vi "Stage Motion Sub VI.vi"() -> ()   [LabVIEW 2009]
uses:
  <vilib>/Instr/_visa.llb/VISA Configure Serial Port (Instr).vi
  <vilib>/Platform/TimedLoop/XDataNode/XDataNode.xnode
  <vilib>/Platform/TimedLoop/XDataNode/loadlvalarms.vi
  <vilib>/Platform/TimedLoop/XDataNode/timing_clust.ctl
  <vilib>/Platform/TimedLoop/XDataNode/nitl_modes.ctl
  <vilib>/Platform/TimedLoop/XDataNode/wakeup.ctl
  <vilib>/Platform/TimedLoop/XDataNode/XDNodeRunTimeDep.lvlib
panel:
  in  "Move to Position 1":bool
  in  "Move to Position 2":bool
  in  "Move to Position 3":bool
  in  "Move to Position 4":bool
  in  "Move to Position 5":bool
  in  "Lower Ch. Cap.":bool
  in  "Dump Beads":bool
  in  "+z":bool
  in  "-z":bool
  in  "z nudge increment (um)":dbl=0.5
  in  "Lower Cap.":bool
  in  "Upper Cap.":bool
  in  "Move to Position":bool
  in  "Set Position":bool
  in  "Position":dbl=1.0 min=1.0 max=10.0 step=1.0
  in  "Saved Stage Positions":dbl[][](array[numeric])=[[1.0, 0.0, 0.0, 0.0], [2.0, 0.0, 0.0, 0.0], [3.0, 0.0, 0.0, 0.0], [4.0, 0.0, 0.0, 0.0], [5.0, 0.0, 0.0, 0.0], [6.0, 0.0, 0.0, 0.0], [7.0, 0.0, 0.0, 0.0], [8.0, 0.0, 0.0, 0.0], [9.0, 0.0, 0.0, 0.0], [10.0, 0.0, 0.0, 0.0]]
  in  "Set Position 1":bool
  in  "Set Position 2":bool
  in  "Set Position 3":bool
  in  "Set Position 4":bool
  in  "Set Position 5":bool
  in  "Position Label 5":string="Lower Channel Cap" caption="5"
  out "Stage Moving":bool
  out "Stage Control Serial Error":errorcluster
  in  "Sample Chamber Stage Serial Port":refnum<visa-resource-name>="ChamberStageCOM4"
  in  "Position 4 Label":string="Dump beads" caption="4"
  in  "Position 3 Label":string="Measurement spot" caption="3"
  in  "Position 2 Label":string="Lower capillary" caption="2"
  in  "Position 1 Label":string="Upper capillary" caption="1"
  in  "Stop All":bool
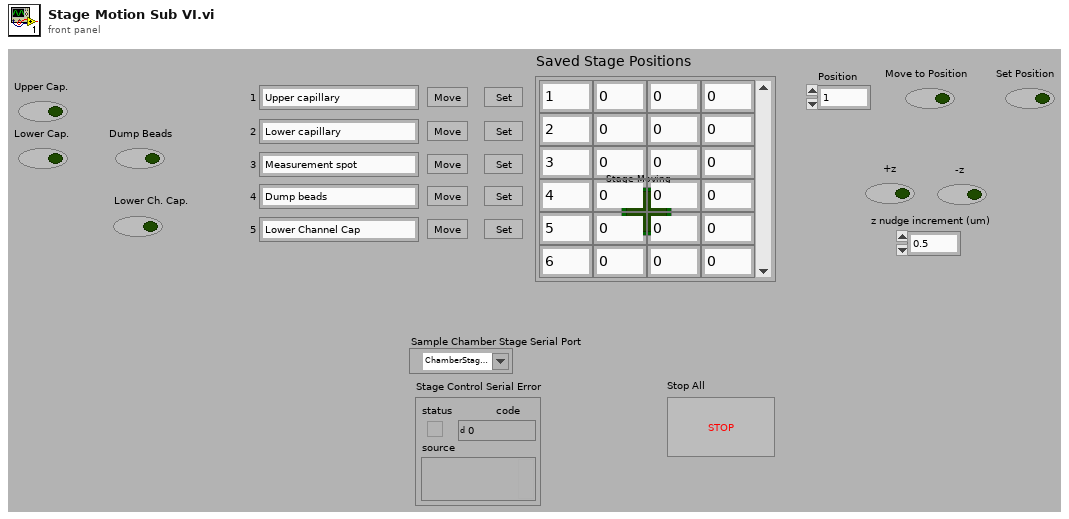
[diagram p1: front panel]
types:
  T1 = typedef "XDNodeRunTimeDep.lvlib/timing_clust.ctl" = cluster{"Expected End [f-1]":u64, "Actual End [f-1]":u64, "Finished Late? [f-1]":bool, "Expected End [i-1]":u64, "Actual End [i-1]":u64, "Finished Late? [i-1]":bool, "Expected Start [i]":u64, "Actual Start [i]":u64, "Expected Start [f]":u64, "Actual Start [f]":u64, "Source Name":string, "Structure Name":string, "Period":i64, "Deadline":i64, "Offset":i64, "Start":i64, "Priority":i32, "Timeout":i32, "Mode":T2, "Wakeup Reason":T3, "Error":errorcluster, "Source Type":string, "Secondary Source Type":string, "Global End Time":u64, "Global Start Time":u64, "Frame Duration":u64, "Iteration Duration":u64, "Assigned CPU":i32, "I/O Scan Engine Mode":u32}
  T2 = typedef "XDNodeRunTimeDep.lvlib/nitl_modes.ctl" = enum32{"No Change", "Process missed periods, maintain original phase", "Discard missed periods, maintain original phase", "Process missed periods, ignore original phase", "Discard missed periods, ignore original phase"}
  T3 = typedef "XDNodeRunTimeDep.lvlib/wakeup.ctl" = enum32{"Normal", "Aborted", "Asynchronous wakeup", "Timing source error", "Timed loop error", "Timeout"}
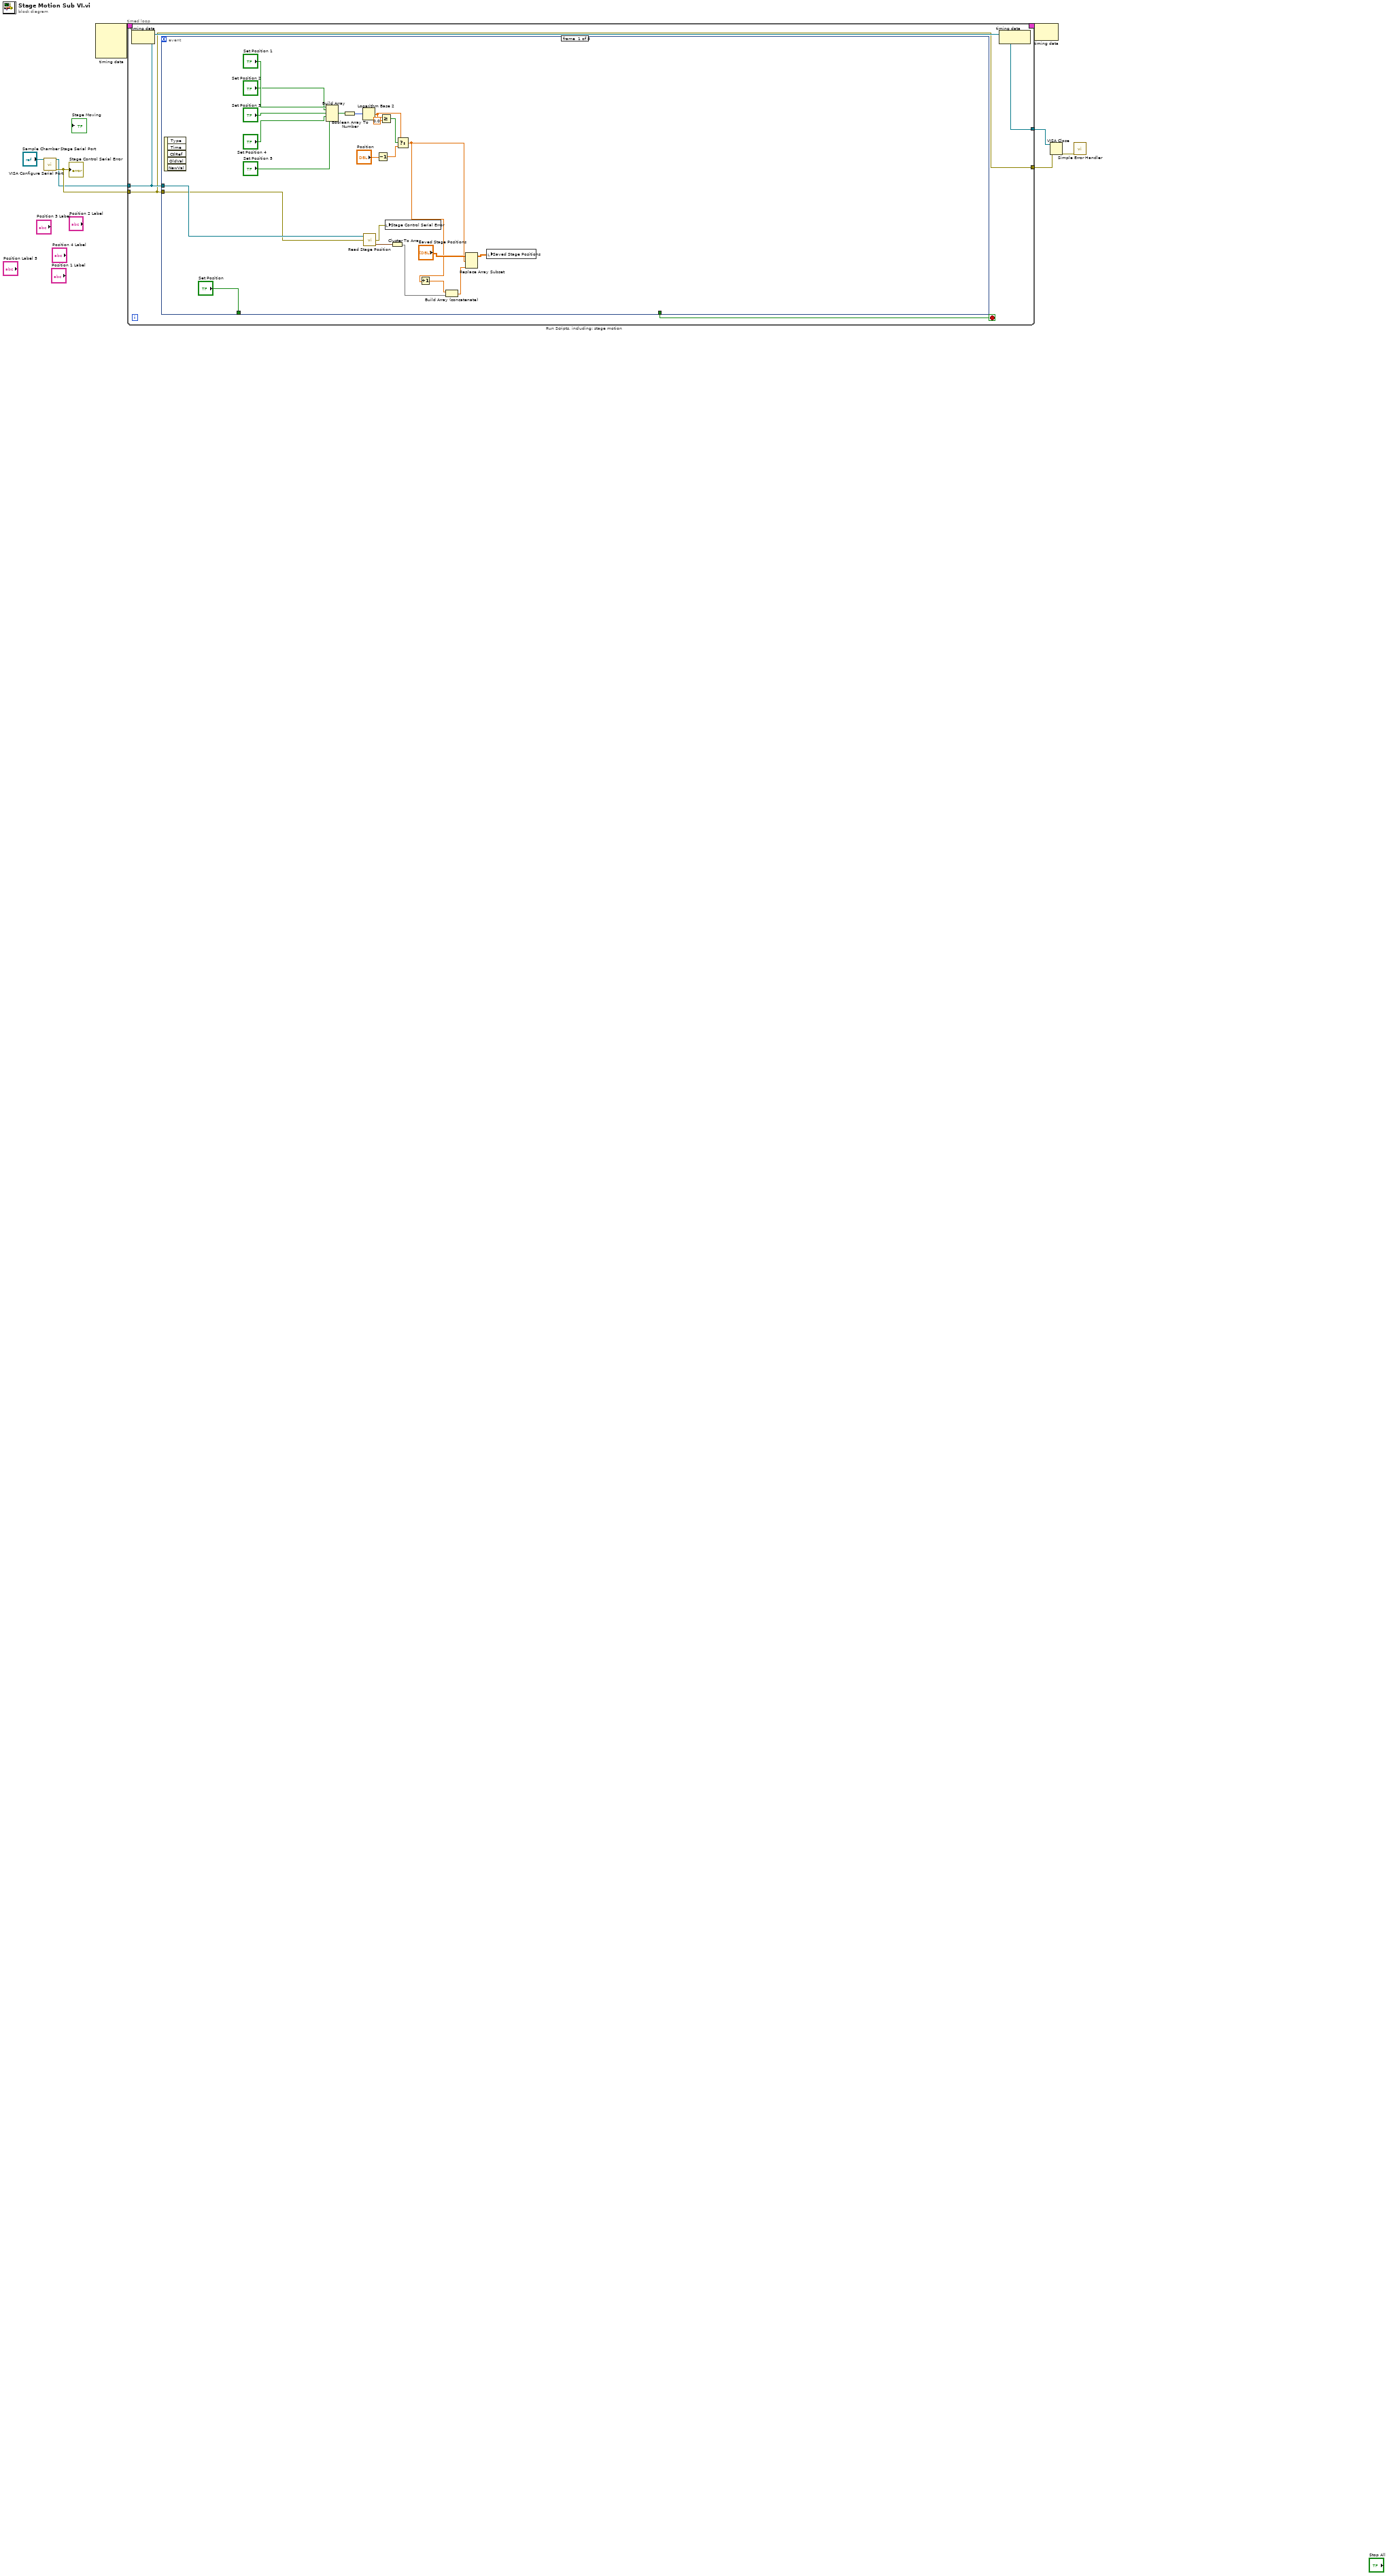
[diagram p0: block diagram]
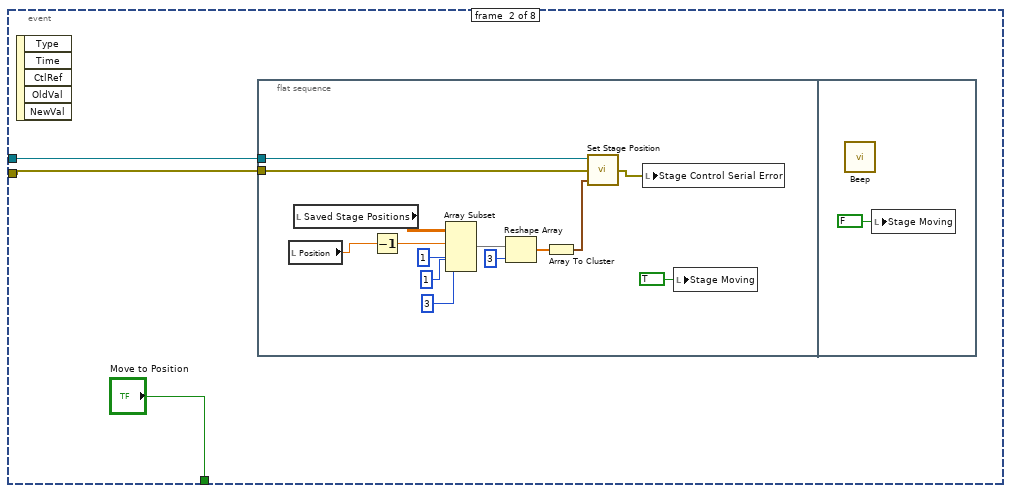
[diagram p2: hidden frame]
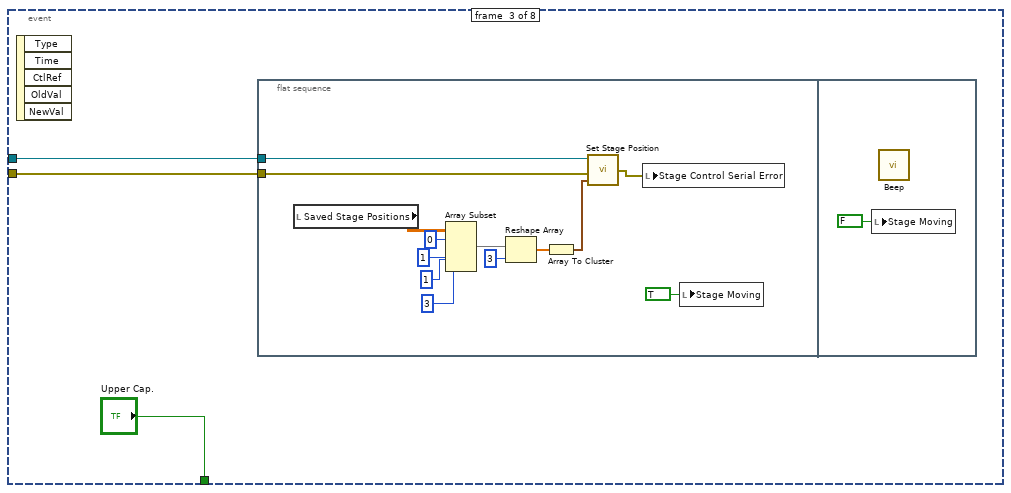
[diagram p3: hidden frame]
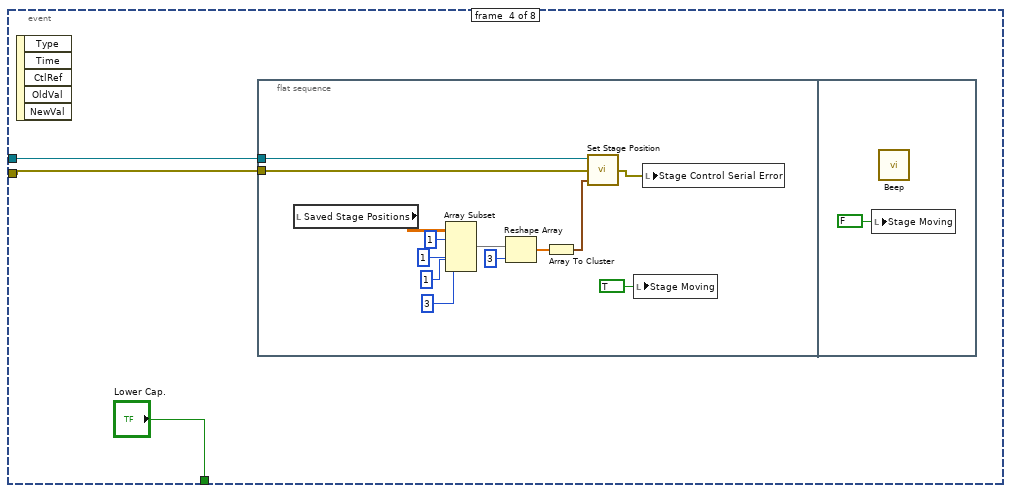
[diagram p4: hidden frame]
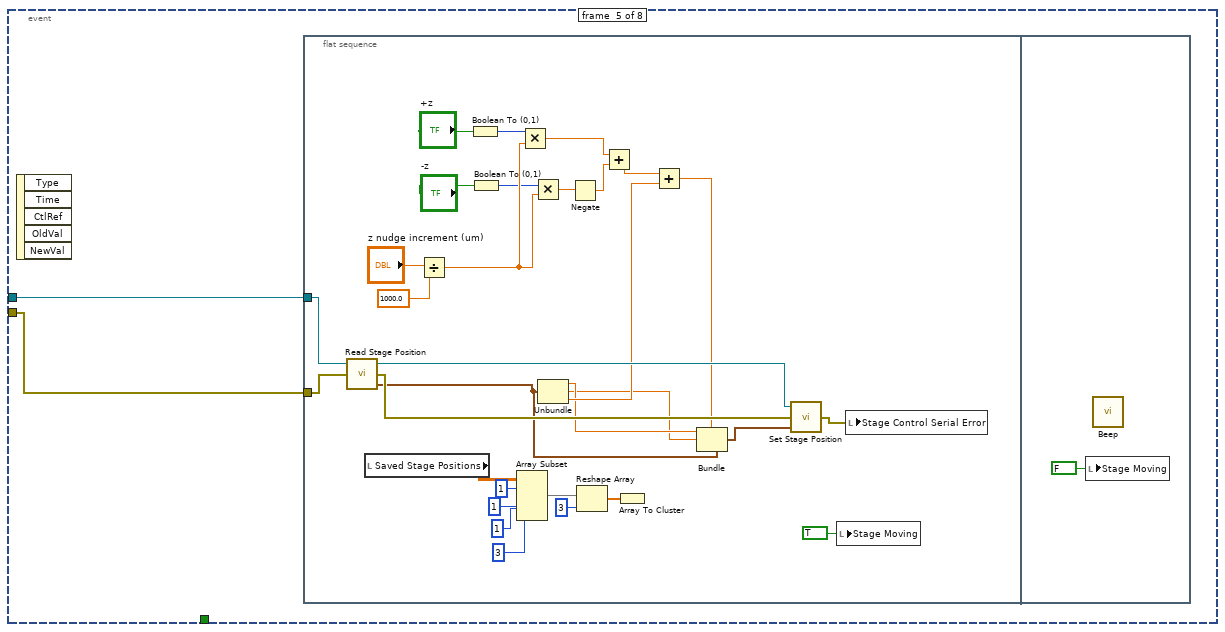
[diagram p5: hidden frame]
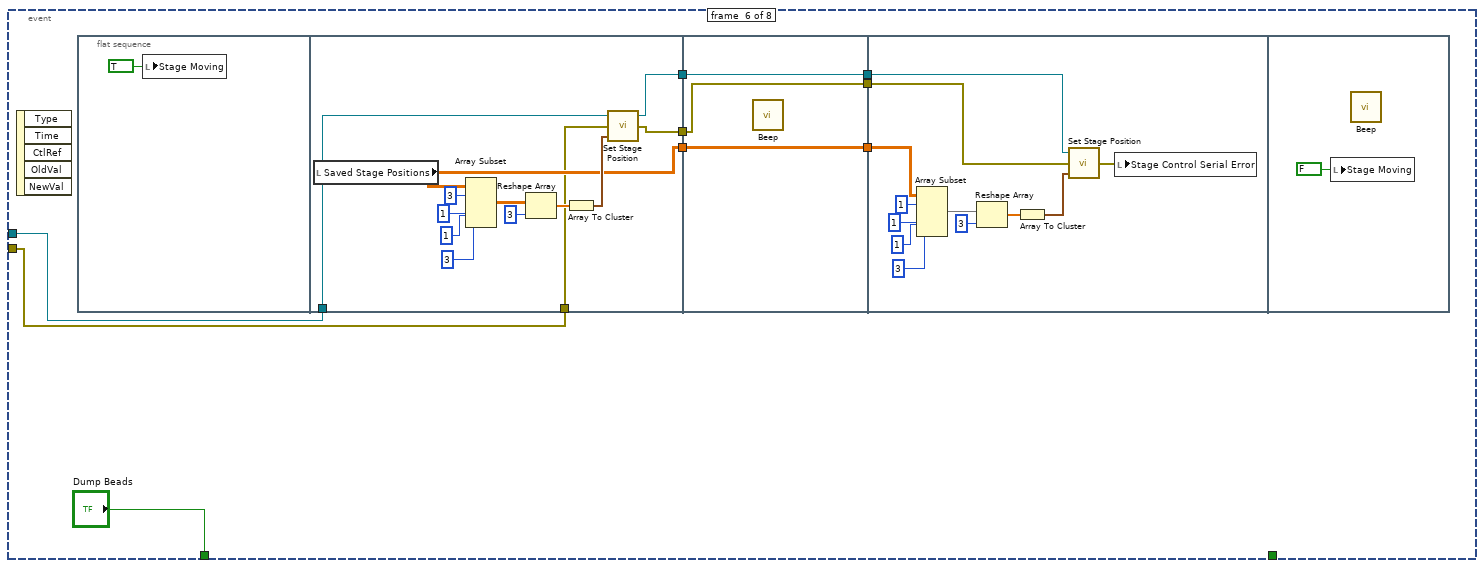
[diagram p6: hidden frame]
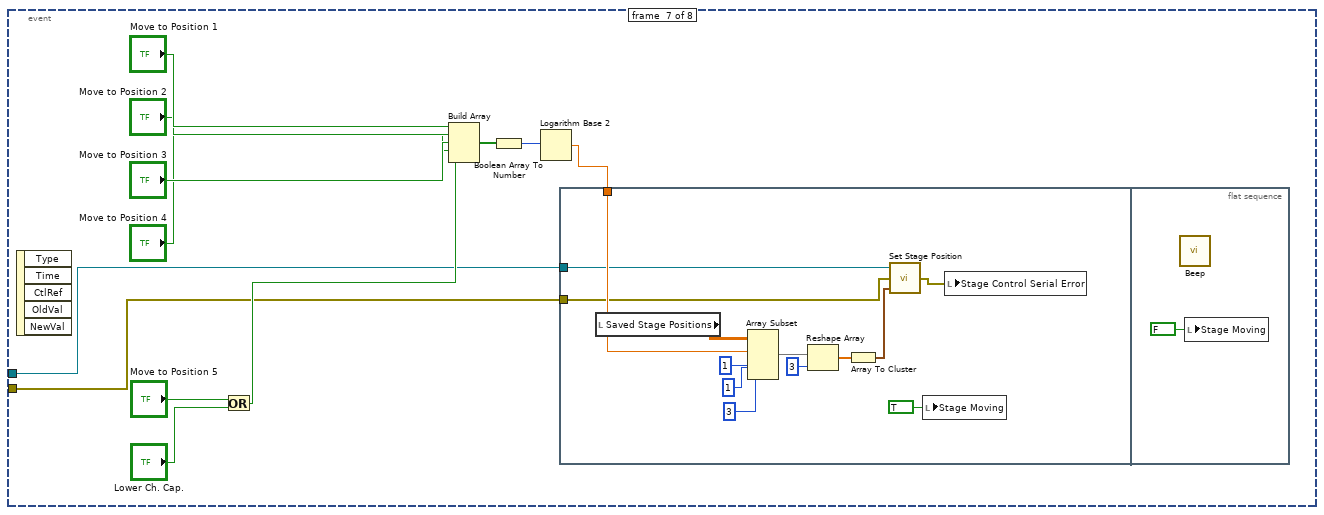
[diagram p7: hidden frame]
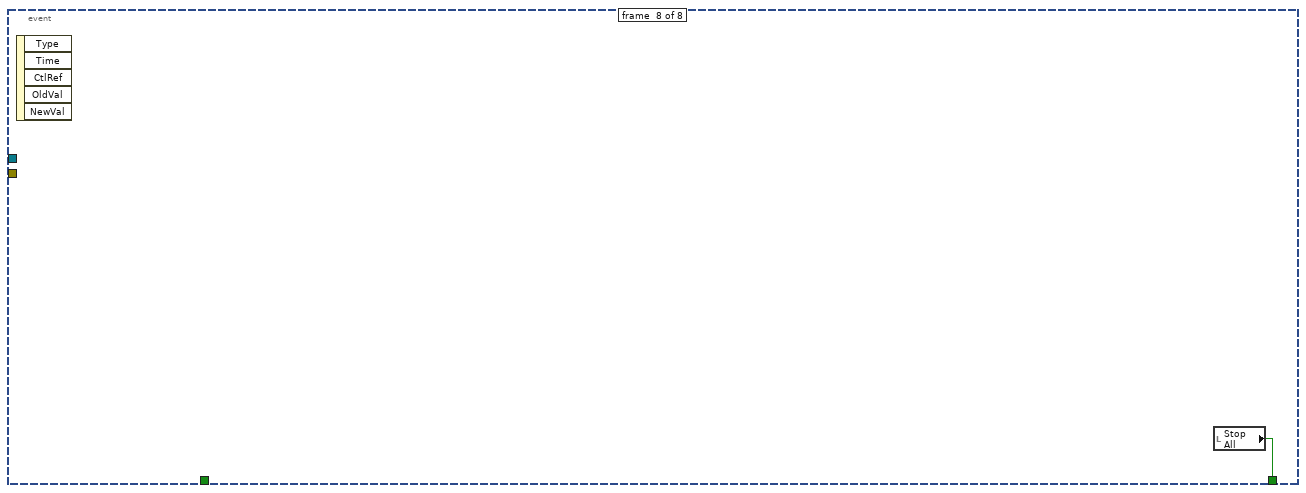
[diagram p8: hidden frame]
diagram:
  n1 = call-poly "VISA Configure Serial Port"("VISA resource name"="Sample Chamber Stage Serial Port") -> ("VISA resource name out"=w3:refnum<visa-resource-name>, "error out"=w4:errorcluster)  [unwired: 5 in, 8 out]
  "Stage Control Serial Error" <- w4
  n2 = node-c288() -> (w8:T1)  [unwired: 4 in]
  n3 = timed-loop "Run Scripts, including: stage motion" {
    tunnel: w4 -> [w9]
    tunnel: w3 -> [w10]
    tunnel: [w10] -> w2
    tunnel: [w9] -> w1
    timing: w8 -> [_]
    timing-out: [_] -> w7
    stop <- w11 stop-if-true
    n4 = node-c288() -> ()  [unwired: 1 in, 1 out]
    n5 = event shown="[7] \"Stop All\": Value Change" {
      selector: _ -> [_ _ _ _ _ _ _ _]
      dyn-events: _ -> [_ _ _ _ _ _ _ _]
      timeout: _ -> [_ _ _ _ _ _ _ _]
      tunnel: ["Set Position" "Move to Position" "Upper Cap." "Lower Cap." _ "Dump Beads" _ _] -> _
      tunnel: [_ _ _ _ _ _ _ w188] -> w11
      tunnel: w9 -> [w29 w37 w55 w72 w89 w123 w162 _]
      tunnel: w10 -> [w30 w38 w56 w73 w90 w124 w163 _]
      event #0 {
        n6 = event-data() -> ()  [unwired: 1 in, 5 out]
        n7 = Build Array("Set Position 1", "Set Position 2", "Set Position 3", "Set Position 4", "Set Position 5") -> (w28:bool[])
        n8 = Boolean Array To Number(Boolean array=w28) -> (number=w27:u32)
        n9 = Logarithm Base 2(1:w27) -> (0:w19:dbl)
        n10 = call "Read Stage Position.vi"("error in"=w29, "VISA resource name in"=w30) -> ("Current Position"=w34:cluster{dbl, dbl, dbl}, "error out"=w33:errorcluster)  [unwired: 2 out]
        n11 = Decrement(x="Position") -> (x-1=w17:dbl)
        n12 = Greater Or Equal?(x=w19, y=0.0) -> (x >= y?=w20:bool)
        n13 = local write "Stage Control Serial Error"(w33) -> ()
        n14 = Cluster To Array(cluster=w34) -> (array=w31:dbl[])
        n15 = Select(t=w19, s=w20, f=w17) -> (s? t:f=w16:dbl)
        n16 = Increment(x=w16) -> (x+1=w15:dbl)
        n17 = Build Array (concatenate)(w15, w31) -> (w14:dbl[])
        n18 = Replace Array Subset(array="Saved Stage Positions", new element=w14, index (row)=w16) -> (w32:dbl[][])  [unwired: 1 in]
        n19 = local write "Saved Stage Positions"(w32) -> ()
      }
      event #1 {
        n20 = event-data() -> ()  [unwired: 1 in, 5 out]
        n21 = flat-sequence {
          tunnel: w38 -> [w41]
          tunnel: w37 -> [w40]
          frame #0 {
            n22 = local read "Position"() -> (w53:dbl)
            n23 = local read "Saved Stage Positions"() -> (w51:dbl[][])
            n24 = Decrement(x=w53) -> (x-1=w50:dbl)
            n25 = Array Subset(array=w51, index (row)=w50, length (row)=1 ("length"), index (col)=1 ("index"), length (col)=3 ("length")) -> (w47:dbl[][])
            n26 = Reshape Array(w47, 3 ("dimension size")) -> (w45:dbl[])
            n27 = Array To Cluster(array=w45) -> (cluster=w44:cluster{"[0]":dbl, "[1]":dbl, "[2]":dbl})
            n28 = call "Set Stage Position.vi"("Position"=w44, "error in"=w40, "VISA resource name in"=w41) -> ("error out"=w43:errorcluster)  [unwired: 2 out]
            n29 = local write "Stage Control Serial Error"(w43) -> ()
            n30 = local write "Stage Moving"(TRUE ("Stage Moving")) -> ()
          }
          frame #1 {
            n31 = call <vilib>:"Beep.vi"() -> ()  [unwired: 3 in, 9 out]
            n32 = local write "Stage Moving"(FALSE ("Stage Moving")) -> ()
          }
        }
      }
      event #2 {
        n33 = event-data() -> ()  [unwired: 1 in, 5 out]
        n34 = flat-sequence {
          tunnel: w56 -> [w59]
          tunnel: w55 -> [w58]
          frame #0 {
            n35 = local read "Saved Stage Positions"() -> (w69:dbl[][])
            n36 = Array Subset(array=w69, index (row)=0 ("index"), length (row)=1 ("length"), index (col)=1 ("index"), length (col)=3 ("length")) -> (w66:dbl[][])
            n37 = Reshape Array(w66, 3 ("dimension size")) -> (w64:dbl[])
            n38 = Array To Cluster(array=w64) -> (cluster=w63:cluster{"[0]":dbl, "[1]":dbl, "[2]":dbl})
            n39 = call "Set Stage Position.vi"("Position"=w63, "error in"=w58, "VISA resource name in"=w59) -> ("error out"=w62:errorcluster)  [unwired: 2 out]
            n40 = local write "Stage Control Serial Error"(w62) -> ()
            n41 = local write "Stage Moving"(TRUE ("Stage Moving")) -> ()
          }
          frame #1 {
            n42 = local write "Stage Moving"(FALSE ("Stage Moving")) -> ()
            n43 = call <vilib>:"Beep.vi"() -> ()  [unwired: 3 in, 9 out]
          }
        }
      }
      event #3 {
        n44 = event-data() -> ()  [unwired: 1 in, 5 out]
        n45 = flat-sequence {
          tunnel: w73 -> [w76]
          tunnel: w72 -> [w75]
          frame #0 {
            n46 = local read "Saved Stage Positions"() -> (w86:dbl[][])
            n47 = Array Subset(array=w86, index (row)=1 ("index"), length (row)=1 ("length"), index (col)=1 ("index"), length (col)=3 ("length")) -> (w83:dbl[][])
            n48 = Reshape Array(w83, 3 ("dimension size")) -> (w81:dbl[])
            n49 = Array To Cluster(array=w81) -> (cluster=w80:cluster{"[0]":dbl, "[1]":dbl, "[2]":dbl})
            n50 = call "Set Stage Position.vi"("Position"=w80, "error in"=w75, "VISA resource name in"=w76) -> ("error out"=w79:errorcluster)  [unwired: 2 out]
            n51 = local write "Stage Moving"(TRUE ("Stage Moving")) -> ()
            n52 = local write "Stage Control Serial Error"(w79) -> ()
          }
          frame #1 {
            n53 = local write "Stage Moving"(FALSE ("Stage Moving")) -> ()
            n54 = call <vilib>:"Beep.vi"() -> ()  [unwired: 3 in, 9 out]
          }
        }
      }
      event #4 {
        n55 = event-data() -> ()  [unwired: 1 in, 5 out]
        n56 = flat-sequence {
          tunnel: w89 -> [w111]
          tunnel: w90 -> [w91]
          frame #0 {
            n57 = call "Read Stage Position.vi"("error in"=w111, "VISA resource name in"=w91) -> ("Current Position"=w96:cluster{dbl, dbl, dbl}, "error out"=w109:errorcluster, "VISA resource name out"=w110:refnum<visa-resource-name>)  [unwired: 1 out]
            n58 = local read "Saved Stage Positions"() -> (w120:dbl[][])
            n59 = Divide(x="z nudge increment (um)", y=1000.0) -> (x/y=w108:dbl)
            n60 = Boolean To (0,1)(Boolean="+z") -> (0, 1=w100:i16)
            n61 = Boolean To (0,1)(Boolean="-z") -> (0, 1=w101:i16)
            n62 = Array Subset(array=w120, index (row)=1 ("index"), length (row)=1 ("length"), index (col)=1 ("index"), length (col)=3 ("length")) -> (w117:dbl[][])
            n63 = Multiply(x=w100, y=w108) -> (x*y=w104:dbl)
            n64 = Multiply(x=w101, y=w108) -> (x*y=w102:dbl)
            n65 = Unbundle(w96) -> (w94:dbl, w93:dbl, w97:dbl)
            n66 = Negate(x=w102) -> (-x=w103:dbl)
            n67 = Reshape Array(w117, 3 ("dimension size")) -> (w115:dbl[])
            n68 = Add(x=w104, y=w103) -> (x+y=w105:dbl)
            n69 = Array To Cluster(array=w115) -> ()  [unwired: 1 out]
            n70 = Add(x=w105, y=w97) -> (x+y=w95:dbl)
            n71 = Bundle(cluster=w96, w94, w93, w95) -> (w92:cluster{dbl, dbl, dbl})
            n72 = call "Set Stage Position.vi"("Position"=w92, "error in"=w109, "VISA resource name in"=w110) -> ("error out"=w114:errorcluster)  [unwired: 2 out]
            n73 = local write "Stage Moving"(TRUE ("Stage Moving")) -> ()
            n74 = local write "Stage Control Serial Error"(w114) -> ()
          }
          frame #1 {
            n75 = local write "Stage Moving"(FALSE ("Stage Moving")) -> ()
            n76 = call <vilib>:"Beep.vi"() -> ()  [unwired: 3 in, 9 out]
          }
        }
      }
      event #5 {
        n77 = event-data() -> ()  [unwired: 1 in, 5 out]
        n78 = flat-sequence {
          tunnel: [w137] -> w129
          tunnel: [w136] -> w127
          tunnel: [w135] -> w125
          tunnel: w124 -> [w134]
          tunnel: w123 -> [w133]
          tunnel: [w148] -> w130
          tunnel: w129 -> [w148]
          tunnel: [w147] -> w128
          tunnel: w127 -> [w147]
          tunnel: [w146] -> w126
          tunnel: w125 -> [w146]
          tunnel: w130 -> [w152]
          tunnel: w128 -> [w151]
          tunnel: w126 -> [w153]
          frame #0 {
            n79 = local write "Stage Moving"(TRUE ("Stage Moving")) -> ()
          }
          frame #1 {
            n80 = local read "Saved Stage Positions"() -> (w135:dbl[][])
            n81 = Array Subset(array=w135, index (row)=3 ("index"), length (row)=1 ("length"), index (col)=1 ("index"), length (col)=3 ("length")) -> (w142:dbl[][])
            n82 = Reshape Array(w142, 3 ("dimension size")) -> (w140:dbl[])
            n83 = Array To Cluster(array=w140) -> (cluster=w139:cluster{"[0]":dbl, "[1]":dbl, "[2]":dbl})
            n84 = call "Set Stage Position.vi"("Position"=w139, "error in"=w133, "VISA resource name in"=w134) -> ("error out"=w136:errorcluster, "VISA resource name out"=w137:refnum<visa-resource-name>)  [unwired: 1 out]
          }
          frame #2 {
            n85 = call <vilib>:"Beep.vi"() -> ()  [unwired: 3 in, 9 out]
          }
          frame #3 {
            n86 = Array Subset(array=w153, index (row)=1 ("index"), length (row)=1 ("length"), index (col)=1 ("index"), length (col)=3 ("length")) -> (w157:dbl[][])
            n87 = Reshape Array(w157, 3 ("dimension size")) -> (w155:dbl[])
            n88 = Array To Cluster(array=w155) -> (cluster=w150:cluster{"[0]":dbl, "[1]":dbl, "[2]":dbl})
            n89 = call "Set Stage Position.vi"("Position"=w150, "error in"=w151, "VISA resource name in"=w152) -> ("error out"=w149:errorcluster)  [unwired: 2 out]
            n90 = local write "Stage Control Serial Error"(w149) -> ()
          }
          frame #4 {
            n91 = local write "Stage Moving"(FALSE ("Stage Moving")) -> ()
            n92 = call <vilib>:"Beep.vi"() -> ()  [unwired: 3 in, 9 out]
          }
        }
      }
      event #6 {
        n93 = event-data() -> ()  [unwired: 1 in, 5 out]
        n94 = Or(x="Move to Position 5", y="Lower Ch. Cap.") -> (x .or. y?=w165:bool)
        n95 = Build Array("Move to Position 1", "Move to Position 2", "Move to Position 3", "Move to Position 4", w165) -> (w168:bool[])
        n96 = Boolean Array To Number(Boolean array=w168) -> (number=w167:u32)
        n97 = Logarithm Base 2(1:w167) -> (0:w166:dbl)
        n98 = flat-sequence {
          tunnel: w166 -> [w177]
          tunnel: w163 -> [w175]
          tunnel: w162 -> [w174]
          frame #0 {
            n99 = local read "Saved Stage Positions"() -> (w185:dbl[][])
            n100 = Array Subset(array=w185, index (row)=w177, length (row)=1 ("length"), index (col)=1 ("index"), length (col)=3 ("length")) -> (w182:dbl[][])
            n101 = Reshape Array(w182, 3 ("dimension size")) -> (w180:dbl[])
            n102 = Array To Cluster(array=w180) -> (cluster=w179:cluster{"[0]":dbl, "[1]":dbl, "[2]":dbl})
            n103 = call "Set Stage Position.vi"("Position"=w179, "error in"=w174, "VISA resource name in"=w175) -> ("error out"=w178:errorcluster)  [unwired: 2 out]
            n104 = local write "Stage Moving"(TRUE ("Stage Moving")) -> ()
            n105 = local write "Stage Control Serial Error"(w178) -> ()
          }
          frame #1 {
            n106 = call <vilib>:"Beep.vi"() -> ()  [unwired: 3 in, 9 out]
            n107 = local write "Stage Moving"(FALSE ("Stage Moving")) -> ()
          }
        }
      }
      event #7 {
        n108 = event-data() -> ()  [unwired: 1 in, 5 out]
        n109 = local read "Stop All"() -> (w188:bool)
      }
    }
    n110 = node-c288() -> ()  [unwired: 1 in, 1 out]
  }
  n111 = node-c288(w7) -> ()  [unwired: 1 out]
  n112 = VISA Close(VISA resource name=w2, error in (no error)=w1) -> (error out=w6:errorcluster)
  n113 = call <vilib>:"Simple Error Handler.vi"("error in (no error)"=w6) -> ()  [unwired: 1 in, 8 out]
